vi "GlobalAutonVariables.vi"() -> ()   [LabVIEW 2020]
panel:
  in  "BR Desired Position":string[](array[string])
  in  "BR Throttle":string[](array[string])
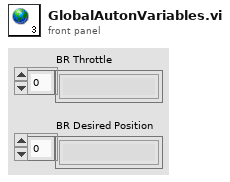
[diagram p1: front panel]
diagram:
